vi "PV Error.vi"(8 "error in (no error)":errorcluster, 9 "Position :":u16=1 min=1 max=10 step=1, 10 "Adress of unit":u16=1 min=1 max=999 step=1, 11 "VISA session":refnum<visa-resource-name>) -> (0 "error out":errorcluster, 1 "Description of error":string, 2 "response (data)":string, 3 "dup VISA session":refnum<visa-resource-name>)   [LabVIEW 2021, in "Pfeiffer Vacuum.lvlib"]
doc: "Read error storage at Position 1 - 10 .\nParameter 360..369\n\nValid Range 1 to 10\nDefault Value: 1"
uses:
  <instrlib>/Pfeiffer Vacuum/Pfeiffer Vacuum.lvlib
panel:
  # "Read error storage at"
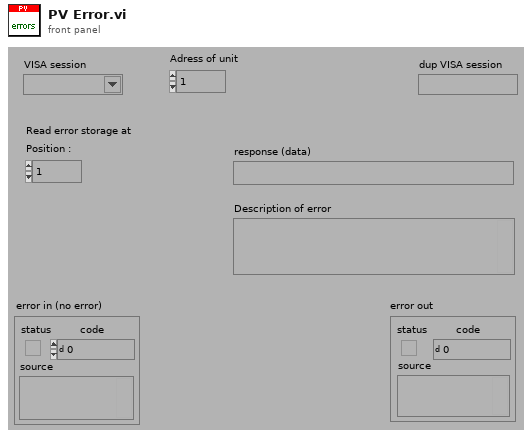
[diagram p1: front panel]
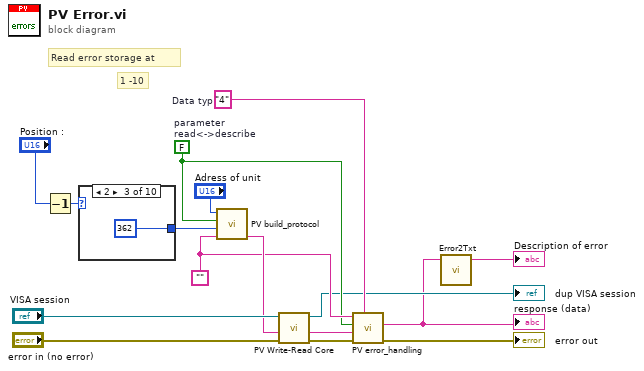
[diagram p0: block diagram]
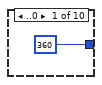
[diagram p2: hidden frame]
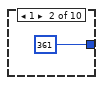
[diagram p3: hidden frame]
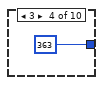
[diagram p4: hidden frame]
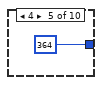
[diagram p5: hidden frame]
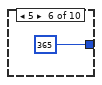
[diagram p6: hidden frame]
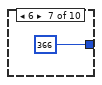
[diagram p7: hidden frame]
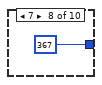
[diagram p8: hidden frame]
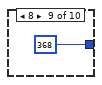
[diagram p9: hidden frame]
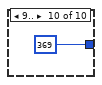
[diagram p10: hidden frame]
diagram:
  w7 = "4"  # Data typ
  w6 = ""
  w5 = FALSE  # parameter read<->describe
  # "1 -10"
  # "Read error storage at"
  n1 = Decrement(x="Position :") -> (x-1=w13:u16)
  n2 = case shown="2" w13 {
    tunnel: [u16 360 ("Parameter-number") u16 361 ("Parameter-number") u16 362 ("Parameter-number") u16 363 ("Parameter-number") u16 364 ("Parameter-number") u16 365 ("Parameter-number") u16 366 ("Parameter-number") u16 367 ("Parameter-number") u16 368 ("Parameter-number") u16 369 ("Parameter-number")] -> w15
    frame ..0 {
    }
    frame 1 {
    }
    frame 2 {
    }
    frame 3 {
    }
    frame 4 {
    }
    frame 5 {
    }
    frame 6 {
    }
    frame 7 {
    }
    frame 8 {
    }
    frame 9.. {
    }
  }
  n3 = call <instrlib>:"PV build_protocol.vi"("Data"=w6, "Parameter-number"=w15, "parameter\nread<->describe"=w5, "Adress"="Adress of unit") -> ("output"=w10:string)  [unwired: 3 in]
  n4 = call <instrlib>:"PV Write-Read Core.vi"("error in"="error in (no error)", "Write data in"=w10, "VISA session"="VISA session") -> ("error out"=w8:errorcluster, "response (data) out"=w9:string, "dup VISA session"=→"dup VISA session":refnum<visa-resource-name>)  [unwired: 2 in]
  n5 = call <instrlib>:"PV error_handling.vi"("Data Typ in"=w7, "error in"=w8, "response (data) in"=w9, "Parameter\nread only<->describe"=w5, "data in"=w6) -> ("error out"=→"error out":errorcluster, "Data out"=w1:string)  [unwired: 4 in, 1 out]
  "response (data)" <- w1
  n6 = call <instrlib>:"Error2Txt.vi"("Error in"=w1) -> ("Description out"=→"Description of error":string)  [unwired: 4 in]
